vi "configEstacion_toArduino_TRASPASO.vi"(8 "error in (no error)":errorcluster, 9 "TRASPASO ASICS INPUT":T1={"COORD X ORIGEN"=0, "COORD  Y ORIGEN"=0, "NºASICS A MOVER"=1, "BANDEJA ORIGEN"=enum."BANDEJA ENTRADA", "BANDEJA DESTINO"=enum."BANDEJA ENTRADA", "COORD X DESTINO "=0, "COORD  Y DESTINO "=0, "CONTEO TRASLADOS"=0}, 10 "Configuracion Estación":T2={"Coordenadas_estacion"={"Coord.Bandeja entrada"={"Coord. X0 entrada"=0, "Coord. Y0 entrada "=0, "Altura Z entrada"=0}, "Coord.Bandeja OK"={"Coord. X0 OK"=0, "Coord. Y0 OK"=0, "Altura Z OK"=0}, "Coord.Bandeja entrada FAIL"={"Coord. X0 FAIL"=0, "Coord. Y0 FAIL"=0, "Altura Z FAIL"=0}, "Coord. Socket"={"Coord. X socket"=0, "Coord. Y socket"=0, "Altura Z socket"=0}}, "Nombre Bandeja"="", "Datos bandeja"={"Nº de columnas "=0, "Nº de filas "=0, "largo"=0, "ancho"=0, "nombre"="nombre", "Paso X (en mm)"=0.0, "Paso Y (en mm)"=0.0, "DISTANCIA SUELO A CHIP  "=0.0, "Nº de celdas totales"=0, "Distancia chips bandejas contiguas"=0.0}}, 11 "VISA resource name":refnum<visa-resource-name>) -> (0 "error IO":errorcluster, 2 "Datos de estación devueltos":string, 3 "trama datos enviada":string)   [LabVIEW 2019]
uses:
  LVPROJ_CONFIG_ESTACION/Type_defs/Coordenadas_estacion.ctl
  LVPROJ_CREAR BANDEJAS/Type_defs/Data_Bandeja.ctl
  TYPE'S DEF/INPUT_TRASPASO_ASICS.ctl
  <vilib>/Utility/error.llb/Error Cluster From Error Code.vi
  <vilib>/ErrorRing/Error Ring.xnode
  SHARED VI'S/SHARED VI'S.lvlib
panel:
  out "return count":u32
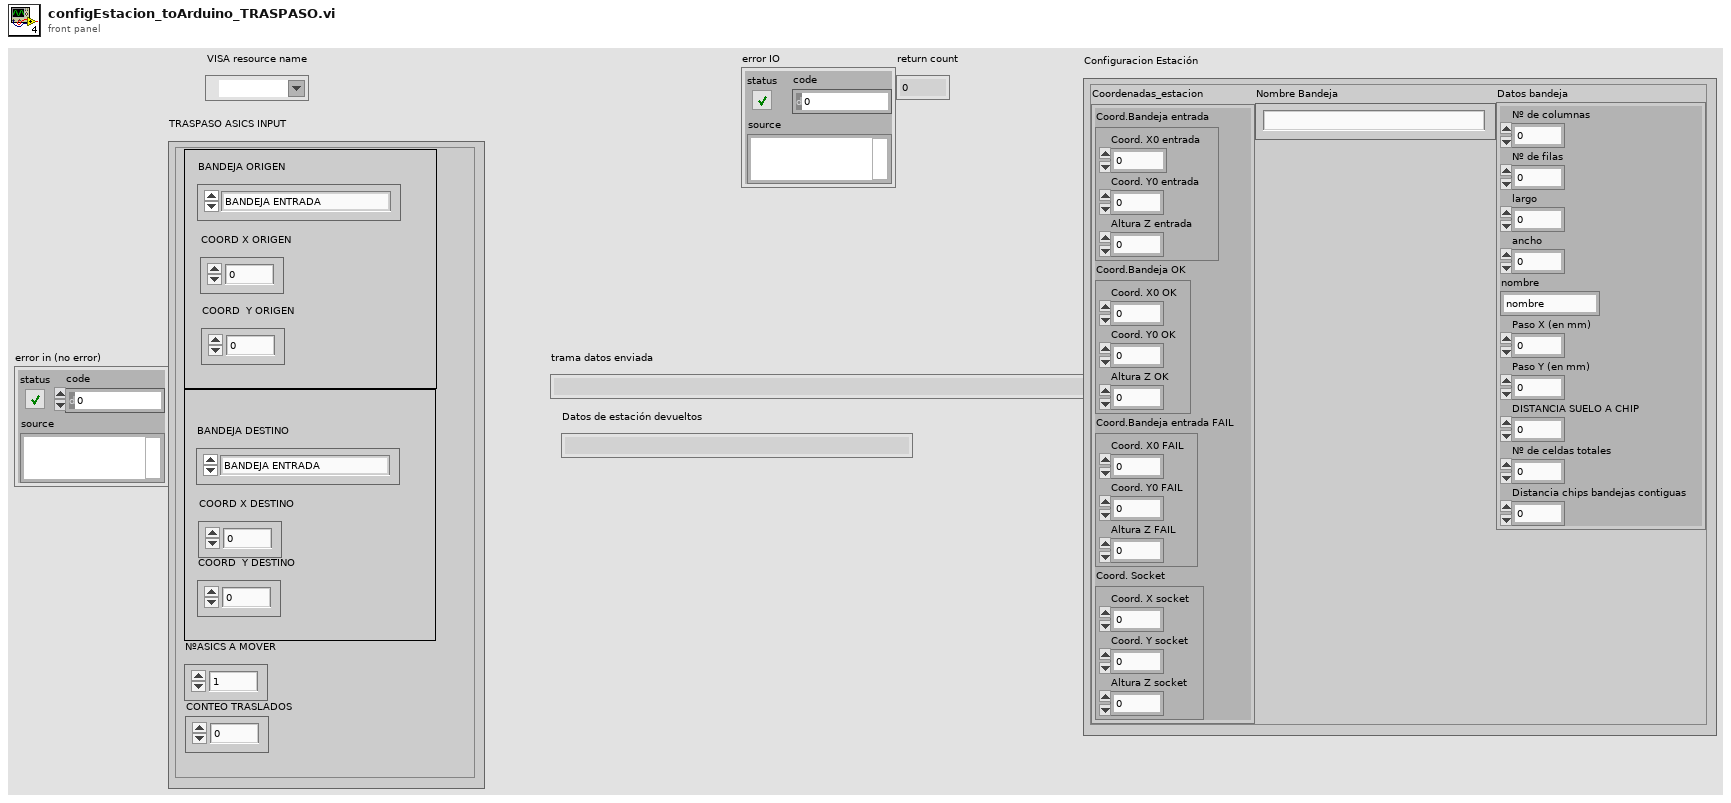
[diagram p1: front panel]
types:
  T1 = typedef "INPUT_TRASPASO_ASICS.ctl" = cluster{"COORD X ORIGEN":u32, "COORD  Y ORIGEN":u32, "NºASICS A MOVER":u32, "BANDEJA ORIGEN":enum16{"BANDEJA ENTRADA", "BANDEJA OK", "BANDEJA NOK"}, "BANDEJA DESTINO":enum16{"BANDEJA ENTRADA", "BANDEJA OK", "BANDEJA NOK"}, "COORD X DESTINO ":u32, "COORD  Y DESTINO ":u32, "CONTEO TRASLADOS":u32}
  T2 = typedef "Configuracion_estación.ctl" = cluster{"Coordenadas_estacion":T3, "Nombre Bandeja":string, "Datos bandeja":T4}
  T3 = typedef "Coordenadas_estacion.ctl" = cluster{"Coord.Bandeja entrada":cluster{"Coord. X0 entrada":u32, "Coord. Y0 entrada ":u32, "Altura Z entrada":u32}, "Coord.Bandeja OK":cluster{"Coord. X0 OK":u32, "Coord. Y0 OK":u32, "Altura Z OK":u32}, "Coord.Bandeja entrada FAIL":cluster{"Coord. X0 FAIL":u32, "Coord. Y0 FAIL":u32, "Altura Z FAIL":u32}, "Coord. Socket":cluster{"Coord. X socket":u32, "Coord. Y socket":u32, "Altura Z socket":u32}}
  T4 = typedef "Data_Bandeja.ctl" = cluster{"Nº de columnas ":u32, "Nº de filas ":u32, "largo":u32, "ancho":u32, "nombre":string, "Paso X (en mm)":dbl, "Paso Y (en mm)":dbl, "DISTANCIA SUELO A CHIP  ":dbl, "Nº de celdas totales":u16, "Distancia chips bandejas contiguas":dbl}
  T5 = enum16{"BANDEJA ENTRADA", "BANDEJA OK", "BANDEJA NOK"}
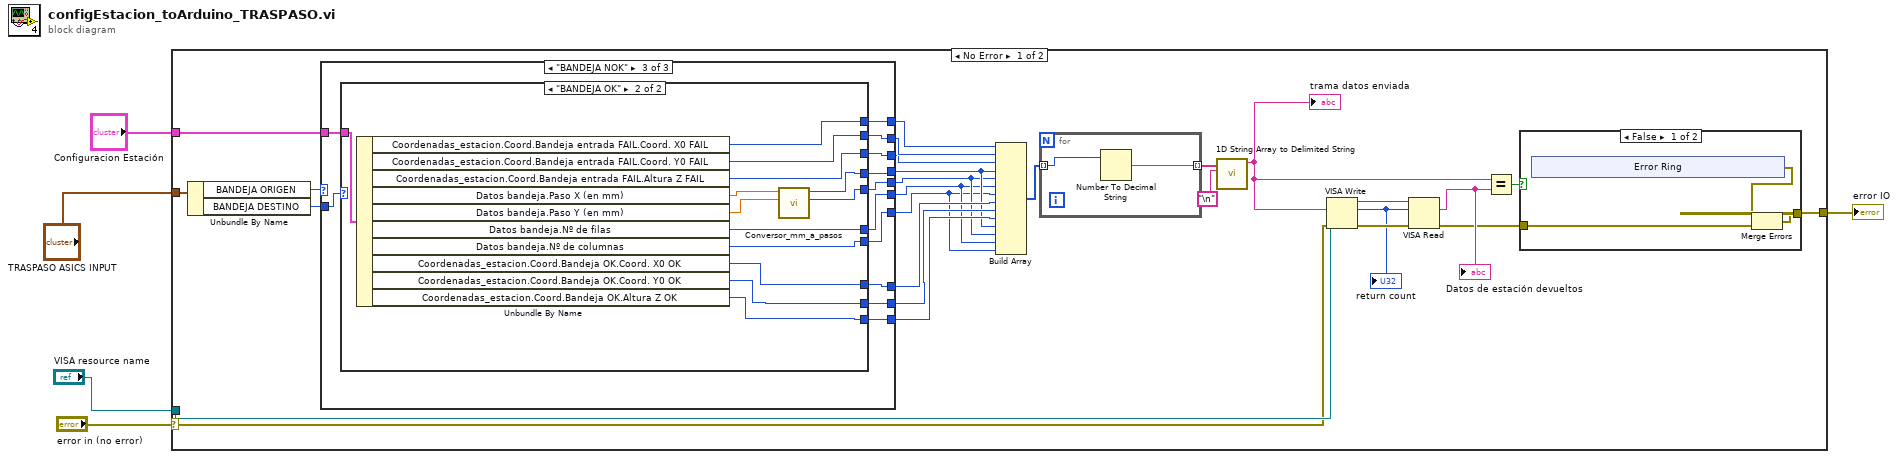
[diagram p0: block diagram]
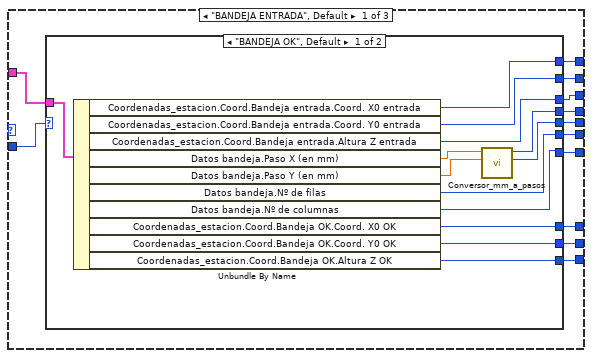
[diagram p2: hidden frame]
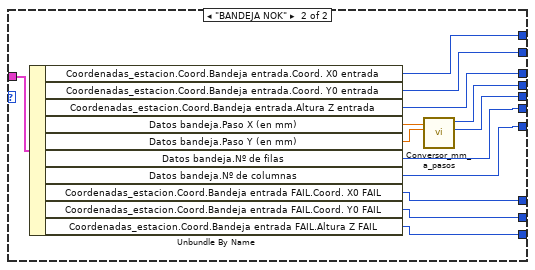
[diagram p3: hidden frame]
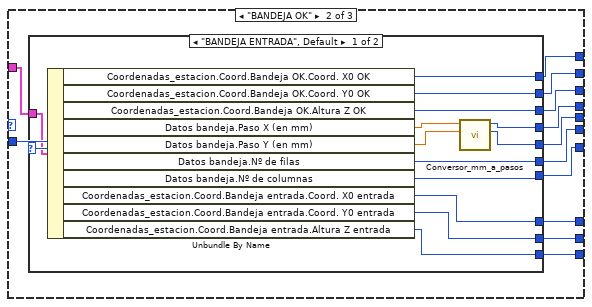
[diagram p4: hidden frame]
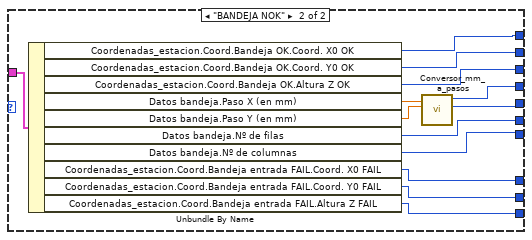
[diagram p5: hidden frame]
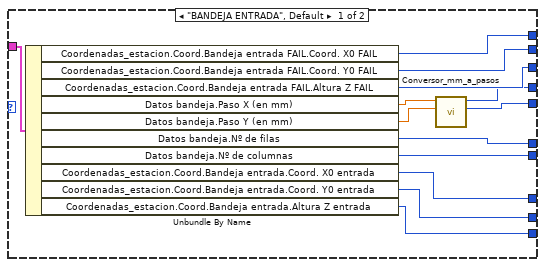
[diagram p6: hidden frame]
diagram:
  n1 = case shown="No Error" "error in (no error)" {
    selector: "error in (no error)" -> [w28 w158]
    tunnel: "Configuracion Estación" -> [w17 _]
    tunnel: "VISA resource name" -> [w29 _]
    tunnel: [w21 w158] -> w2
    tunnel: "TRASPASO ASICS INPUT" -> [w19 _]
    frame No Error {
      n2 = Unbundle By Name(w19) -> ("BANDEJA ORIGEN"=w18:T5, "BANDEJA DESTINO"=w13:T5)
      n3 = case shown="\"BANDEJA NOK\"" w18 {
        tunnel: w17 -> [w43 w81 w119]
        tunnel: [w42 w80 w118] -> w16
        tunnel: [w41 w79 w117] -> w15
        tunnel: [w40 w78 w116] -> w14
        tunnel: w13 -> [w44 w82 w120]
        tunnel: [w39 w71 w115] -> w10
        tunnel: [w38 w73 w113] -> w12
        tunnel: [w37 w72 w114] -> w11
        tunnel: [w36 w77 w112] -> w9
        tunnel: [w35 w76 w111] -> w8
        tunnel: [w34 w75 w110] -> w7
        tunnel: [w33 w74 w109] -> w6
        frame "BANDEJA ENTRADA", Default {
          n4 = case shown="\"BANDEJA OK\", Default" w44 {
            tunnel: w43 -> [w54 w70]
            tunnel: [w57 w69] -> w42
            tunnel: [w56 w68] -> w41
            tunnel: [w55 w67] -> w40
            tunnel: [w51 w64] -> w36
            tunnel: [w50 w63] -> w35
            tunnel: [w49 w62] -> w34
            tunnel: [w48 w61] -> w33
            tunnel: [w47 w60] -> w38
            tunnel: [w46 w59] -> w37
            tunnel: [w45 w58] -> w39
            frame "BANDEJA OK", Default {
              n5 = Unbundle By Name(w54) -> ("Coordenadas_estacion.Coord.Bandeja entrada.Coord. X0 entrada"=w57:u32, "Coordenadas_estacion.Coord.Bandeja entrada.Coord. Y0 entrada"=w56:u32, "Coordenadas_estacion.Coord.Bandeja entrada.Altura Z entrada"=w55:u32, "Datos bandeja.Paso X (en mm)"=w53:dbl, "Datos bandeja.Paso Y (en mm)"=w52:dbl, "Datos bandeja.Nº de filas"=w49:u32, "Datos bandeja.Nº de columnas"=w48:u32, "Coordenadas_estacion.Coord.Bandeja OK.Coord. X0 OK"=w47:u32, "Coordenadas_estacion.Coord.Bandeja OK.Coord. Y0 OK"=w46:u32, "Coordenadas_estacion.Coord.Bandeja OK.Altura Z OK"=w45:u32)
              n6 = call "Conversor_mm_a_pasos.vi"("pasosY"=w52, "pasosX"=w53) -> ("PASOS EN Y"=w50:u32, "PASOS EN X"=w51:u32)  [unwired: 6 in, 2 out]
            }
            frame "BANDEJA NOK" {
              n7 = Unbundle By Name(w70) -> ("Coordenadas_estacion.Coord.Bandeja entrada.Coord. X0 entrada"=w69:u32, "Coordenadas_estacion.Coord.Bandeja entrada.Coord. Y0 entrada"=w68:u32, "Coordenadas_estacion.Coord.Bandeja entrada.Altura Z entrada"=w67:u32, "Datos bandeja.Paso X (en mm)"=w66:dbl, "Datos bandeja.Paso Y (en mm)"=w65:dbl, "Datos bandeja.Nº de filas"=w62:u32, "Datos bandeja.Nº de columnas"=w61:u32, "Coordenadas_estacion.Coord.Bandeja entrada FAIL.Coord. X0 FAIL"=w60:u32, "Coordenadas_estacion.Coord.Bandeja entrada FAIL.Coord. Y0 FAIL"=w59:u32, "Coordenadas_estacion.Coord.Bandeja entrada FAIL.Altura Z FAIL"=w58:u32)
              n8 = call "Conversor_mm_a_pasos.vi"("pasosY"=w65, "pasosX"=w66) -> ("PASOS EN Y"=w63:u32, "PASOS EN X"=w64:u32)  [unwired: 6 in, 2 out]
            }
          }
        }
        frame "BANDEJA OK" {
          n9 = case shown="\"BANDEJA ENTRADA\", Default" w82 {
            tunnel: w81 -> [w95 w108]
            tunnel: [w94 w107] -> w80
            tunnel: [w93 w106] -> w79
            tunnel: [w92 w105] -> w78
            tunnel: [w89 w102] -> w77
            tunnel: [w88 w101] -> w76
            tunnel: [w87 w100] -> w75
            tunnel: [w86 w99] -> w74
            tunnel: [w85 w98] -> w73
            tunnel: [w84 w97] -> w72
            tunnel: [w83 w96] -> w71
            frame "BANDEJA ENTRADA", Default {
              n10 = Unbundle By Name(w95) -> ("Coordenadas_estacion.Coord.Bandeja OK.Coord. X0 OK"=w94:u32, "Coordenadas_estacion.Coord.Bandeja OK.Coord. Y0 OK"=w93:u32, "Coordenadas_estacion.Coord.Bandeja OK.Altura Z OK"=w92:u32, "Datos bandeja.Paso X (en mm)"=w91:dbl, "Datos bandeja.Paso Y (en mm)"=w90:dbl, "Datos bandeja.Nº de filas"=w87:u32, "Datos bandeja.Nº de columnas"=w86:u32, "Coordenadas_estacion.Coord.Bandeja entrada.Coord. X0 entrada"=w85:u32, "Coordenadas_estacion.Coord.Bandeja entrada.Coord. Y0 entrada"=w84:u32, "Coordenadas_estacion.Coord.Bandeja entrada.Altura Z entrada"=w83:u32)
              n11 = call "Conversor_mm_a_pasos.vi"("pasosY"=w90, "pasosX"=w91) -> ("PASOS EN Y"=w88:u32, "PASOS EN X"=w89:u32)  [unwired: 6 in, 2 out]
            }
            frame "BANDEJA NOK" {
              n12 = Unbundle By Name(w108) -> ("Coordenadas_estacion.Coord.Bandeja OK.Coord. X0 OK"=w107:u32, "Coordenadas_estacion.Coord.Bandeja OK.Coord. Y0 OK"=w106:u32, "Coordenadas_estacion.Coord.Bandeja OK.Altura Z OK"=w105:u32, "Datos bandeja.Paso X (en mm)"=w104:dbl, "Datos bandeja.Paso Y (en mm)"=w103:dbl, "Datos bandeja.Nº de filas"=w100:u32, "Datos bandeja.Nº de columnas"=w99:u32, "Coordenadas_estacion.Coord.Bandeja entrada FAIL.Coord. X0 FAIL"=w98:u32, "Coordenadas_estacion.Coord.Bandeja entrada FAIL.Coord. Y0 FAIL"=w97:u32, "Coordenadas_estacion.Coord.Bandeja entrada FAIL.Altura Z FAIL"=w96:u32)
              n13 = call "Conversor_mm_a_pasos.vi"("pasosY"=w103, "pasosX"=w104) -> ("PASOS EN Y"=w101:u32, "PASOS EN X"=w102:u32)  [unwired: 6 in, 2 out]
            }
          }
        }
        frame "BANDEJA NOK" {
          n14 = case shown="\"BANDEJA OK\"" w120 {
            tunnel: w119 -> [w133 w146]
            tunnel: [w132 w145] -> w118
            tunnel: [w131 w144] -> w117
            tunnel: [w130 w143] -> w116
            tunnel: [w122 w135] -> w112
            tunnel: [w121 w134] -> w111
            tunnel: [w129 w142] -> w110
            tunnel: [w128 w141] -> w115
            tunnel: [w127 w140] -> w114
            tunnel: [w126 w139] -> w113
            tunnel: [w125 w138] -> w109
            frame "BANDEJA ENTRADA", Default {
              n15 = Unbundle By Name(w133) -> ("Coordenadas_estacion.Coord.Bandeja entrada FAIL.Coord. X0 FAIL"=w132:u32, "Coordenadas_estacion.Coord.Bandeja entrada FAIL.Coord. Y0 FAIL"=w131:u32, "Coordenadas_estacion.Coord.Bandeja entrada FAIL.Altura Z FAIL"=w130:u32, "Datos bandeja.Paso X (en mm)"=w124:dbl, "Datos bandeja.Paso Y (en mm)"=w123:dbl, "Datos bandeja.Nº de filas"=w129:u32, "Datos bandeja.Nº de columnas"=w125:u32, "Coordenadas_estacion.Coord.Bandeja entrada.Coord. X0 entrada"=w126:u32, "Coordenadas_estacion.Coord.Bandeja entrada.Coord. Y0 entrada"=w127:u32, "Coordenadas_estacion.Coord.Bandeja entrada.Altura Z entrada"=w128:u32)
              n16 = call "Conversor_mm_a_pasos.vi"("pasosY"=w123, "pasosX"=w124) -> ("PASOS EN Y"=w121:u32, "PASOS EN X"=w122:u32)  [unwired: 6 in, 2 out]
            }
            frame "BANDEJA OK" {
              n17 = Unbundle By Name(w146) -> ("Coordenadas_estacion.Coord.Bandeja entrada FAIL.Coord. X0 FAIL"=w145:u32, "Coordenadas_estacion.Coord.Bandeja entrada FAIL.Coord. Y0 FAIL"=w144:u32, "Coordenadas_estacion.Coord.Bandeja entrada FAIL.Altura Z FAIL"=w143:u32, "Datos bandeja.Paso X (en mm)"=w137:dbl, "Datos bandeja.Paso Y (en mm)"=w136:dbl, "Datos bandeja.Nº de filas"=w142:u32, "Datos bandeja.Nº de columnas"=w138:u32, "Coordenadas_estacion.Coord.Bandeja OK.Coord. X0 OK"=w139:u32, "Coordenadas_estacion.Coord.Bandeja OK.Coord. Y0 OK"=w140:u32, "Coordenadas_estacion.Coord.Bandeja OK.Altura Z OK"=w141:u32)
              n18 = call "Conversor_mm_a_pasos.vi"("pasosY"=w136, "pasosX"=w137) -> ("PASOS EN Y"=w134:u32, "PASOS EN X"=w135:u32)  [unwired: 6 in, 2 out]
            }
          }
        }
      }
      n19 = Build Array(w16, w15, w14, w9, w8, w7, w6, w12, w11, w10, w9, w8, w7, w6) -> (w32:u32[])
      n20 = for {
        tunnel: w32 -> [w156] mode=indexing
        tunnel: [w157] -> w31 mode=indexing
        n21 = Number To Decimal String(number=w156) -> (decimal integer string=w157:string)  [unwired: 1 in]
      }
      n22 = call <vilib>:"1D String Array to Delimited String.vi"("delimiter"="\n", "string array"=w31) -> ("delimited string"=w24:string)  [unwired: 9 in]
      "trama datos enviada" <- w24
      n23 = VISA Write(VISA resource name=w29, write buffer=w24, error in (no error)=w28) -> (VISA resource name out=w26:refnum<visa-resource-name>, return count=w25:u32, error out=w27:errorcluster)
      "return count" <- w25
      n24 = VISA Read(VISA resource name=w26, byte count=w25, error in (no error)=w27) -> (read buffer=w23:string, error out=w20:errorcluster)  [unwired: 2 out]
      "Datos de estación devueltos" <- w23
      n25 = Equal?(x=w24, y=w23) -> (x = y?=w22:bool)
      n26 = case shown="False" w22 {
        tunnel: [w149 w155] -> w21
        tunnel: w20 -> [w147 w155]
        frame False {
          n27 = xnode "Error Ring"() -> ("error out"=w148:errorcluster)
          n28 = Merge Errors(w148, w147) -> (w149:errorcluster)
        }
        frame True {
        }
      }
    }
    frame Error {
    }
  }
  "error IO" <- w2
